vi "draw.vi"(0 "reference":refnum<class "AbstractEdge.lvclass">, 1 "graphics":refnum<class "Graphics.lvclass">, 5 "error in (no error)":errorcluster) -> (14 "reference out":refnum<class "AbstractEdge.lvclass">, 19 "error out":errorcluster)   [LabVIEW 2014, in "AbstractEdge.lvclass"]
uses:
  <resource>/Framework/Providers/Open_GDS/UML/AbstractEdge_class/AbstractEdge.lvclass
  <resource>/Framework/Providers/Open_GDS/UML/Graphics_class/Graphics.lvclass
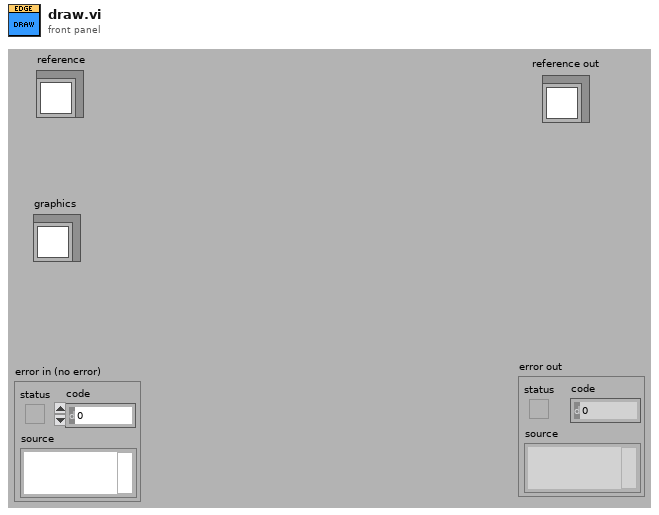
[diagram p1: front panel]
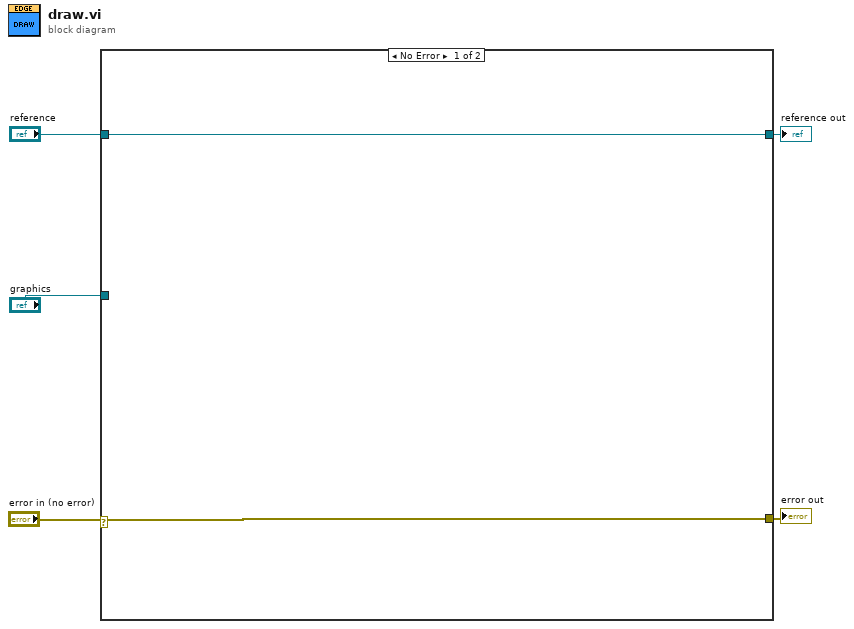
[diagram p0: block diagram]
diagram:
  n1 = case shown="No Error" "error in (no error)" {
    selector: "error in (no error)" -> [w6 w8]
    tunnel: "reference" -> [w7 w9]
    tunnel: [w6 w8] -> w4
    tunnel: [w7 w9] -> w3
    tunnel: "graphics" -> [_ _]
    frame No Error {
    }
    frame Error {
    }
  }
  "reference out" <- w3
  "error out" <- w4
